vi "Server 2 - Copy1.vi"() -> ()   [LabVIEW 2017]
panel:
  out "digit?":bool
  out "Array":dbl[](array[numeric])
  out "data out 2":string
  out "data out":string
  in  "stop":bool
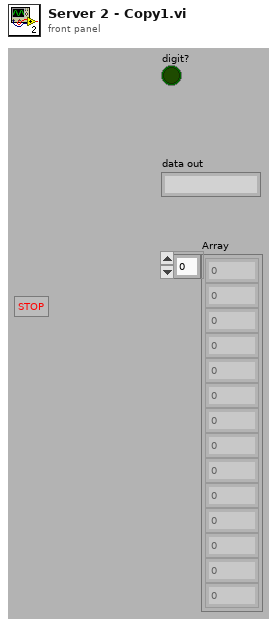
[diagram p1: front panel]
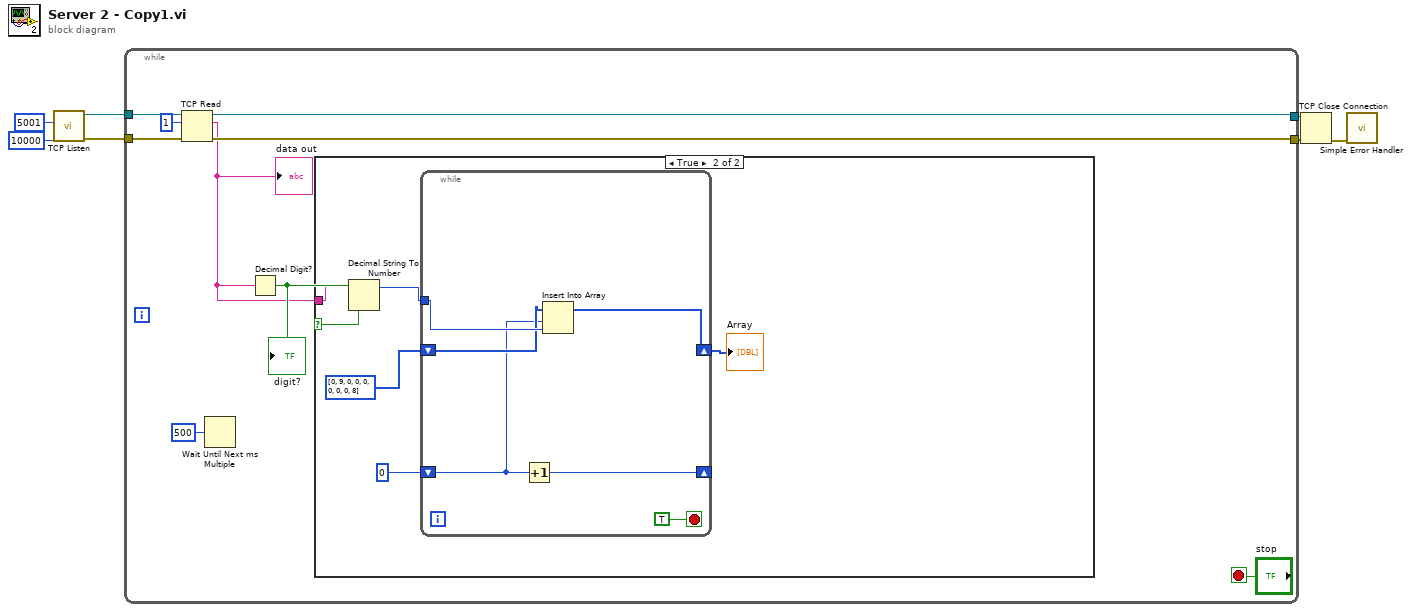
[diagram p0: block diagram]
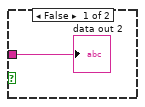
[diagram p2: hidden frame]
diagram:
  n1 = call <vilib>:"TCP Listen.vi"("timeout ms (wait forever: -1)"=10000, "port"=u16 5001) -> ("error out"=w6:errorcluster, "connection ID"=w7:refnum<k5>)  [unwired: 5 in, 3 out]
  n2 = while {
    tunnel: w7 -> [w15]
    tunnel: w6 -> [w14]
    tunnel: [w12] -> w5
    tunnel: [w10] -> w4
    stop <- "stop" stop-if-true
    n3 = TCP Read(connection ID=w15, bytes to read=1, error in (no error)=w14) -> (connection ID out=w12:refnum<k5>, data out=w8:string, error out=w10:errorcluster)  [unwired: 2 in]
    "data out" <- w8
    n4 = Wait Until Next ms Multiple(millisecond multiple=u32 500) -> ()  [unwired: 1 out]
    n5 = Decimal Digit?(1:w8) -> (0:w9:bool)
    "digit?" <- w9
    n6 = case shown="True" w9 {
      tunnel: w8 -> [w17 w19]
      frame False {
        "data out 2" <- w17
      }
      frame True {
        n7 = Decimal String To Number(string=w19) -> (offset past number=w22:i32)  [unwired: 2 in, 1 out]
        n8 = while {
          tunnel: w22 -> [w28]
          shift-right: [w27] -> w20
          shift-left: i32[] [0, 9, 0, 0, 0, 0, 0, 0, 8] -> [w25]
          shift-right: [w24] -> _
          shift-left: 0 -> [w23]
          stop <- TRUE stop-if-true
          n9 = Increment(x=w23) -> (x+1=w24:i32)
          n10 = Insert Into Array(array=w25, index=w23, new element=w28) -> (w27:i32[])
        }
        "Array" <- w20
      }
    }
  }
  n11 = TCP Close Connection(connection ID=w5, error in (no error)=w4) -> (error out=w3:errorcluster)  [unwired: 1 in, 1 out]
  n12 = call <vilib>:"Simple Error Handler.vi"("error in (no error)"=w3) -> ()  [unwired: 4 in, 5 out]
